vi "AcquireMouseInput.vi"() -> ()   [LabVIEW 2019]
uses:
  <vilib>/Utility/inputDevices.llb/mouseAcquire.vi
  <vilib>/Utility/inputDevices.llb/closeMouse.vi
panel:
  in  "Stop Button":bool
  out "Axis Info":T1
  out "Button Info":T2
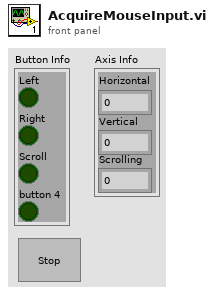
[diagram p1: front panel]
types:
  T1 = cluster{"Horizontal":i32, "Vertical":i32, "Scrolling":i32}
  T2 = cluster{"Left":bool, "Right":bool, "Scroll":bool, "button 4":bool}
  T3 = cluster{"button 1":bool, "button 2":bool, "button 3":bool, "button 4":bool}
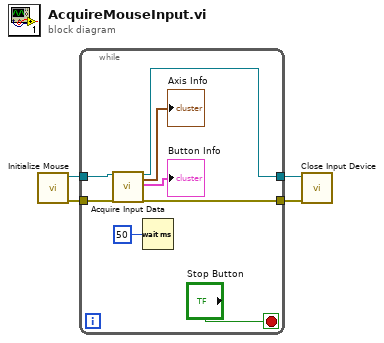
[diagram p0: block diagram]
diagram:
  n1 = call <vilib>:"Initialize Mouse.vi"() -> ("error out"=w3:errorcluster, "device ID"=w4:refnum<k1>)  [unwired: 10 in]
  n2 = while {
    tunnel: w4 -> [w10]
    tunnel: w3 -> [w11]
    tunnel: [w6] -> w2
    tunnel: [w5] -> w1
    stop <- "Stop Button" stop-if-true
    n3 = call-poly <vilib>:"Acquire Input Data.vi"("device ID"=w10, "error in (no error)"=w11) -> ("device ID"=w6:refnum<k1>, "axis info"=→"Axis Info":T1, "button info"=→"Button Info":T3, "error out"=w5:errorcluster)  [unwired: 14 in]
    n4 = Wait (ms)(milliseconds to wait=u32 50) -> ()  [unwired: 1 out]
  }
  n5 = call-poly <vilib>:"Close Input Device.vi"("error in (no error)"=w1, "device ID"=w2) -> ()  [unwired: 8 in, 1 out]
